vi "process data.vi"(0 "waveform array":waveform(dbl)[](array[waveform]), 11 "error in":errorcluster) -> (4 "device 1":cluster{"V":dbl, "dV":dbl, "Q":dbl, "dQ":dbl}, 6 "device 2":cluster{"V":dbl, "dV":dbl, "Q":dbl, "dQ":dbl}, 15 "error out":errorcluster)   [LabVIEW 2026]
uses:
  <vilib>/Utility/error.llb/Error Cluster From Error Code.vi
  <vilib>/ErrorRing/Error Ring.xnode
  <vilib>/Analysis/NI_AALBase.lvlib
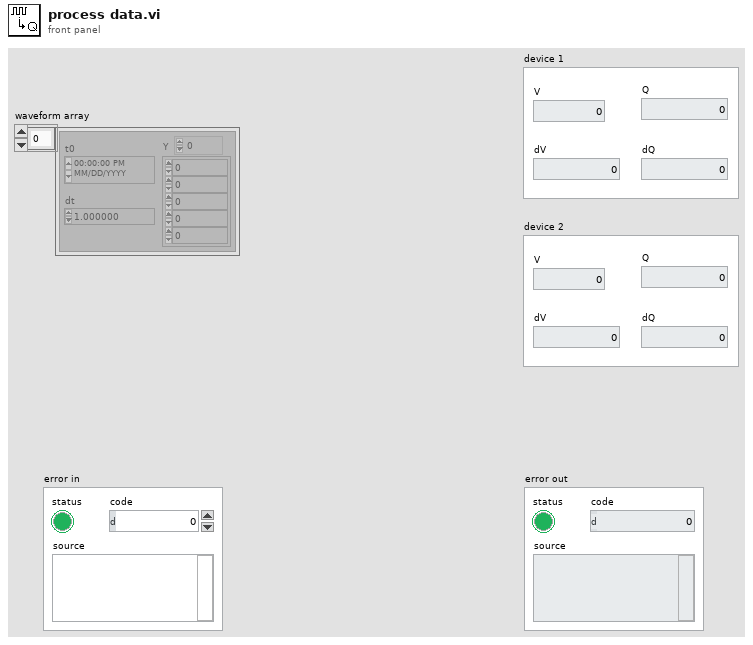
[diagram p1: front panel]
types:
  T1 = cluster{"waveform array[0]":waveform(dbl), "waveform array[1]":waveform(dbl), "waveform array[2]":waveform(dbl), "waveform array[3]":waveform(dbl), "waveform array[4]":waveform(dbl), "waveform array[5]":waveform(dbl), "waveform array[6]":waveform(dbl), "waveform array[7]":waveform(dbl), "waveform array[8]":waveform(dbl)}
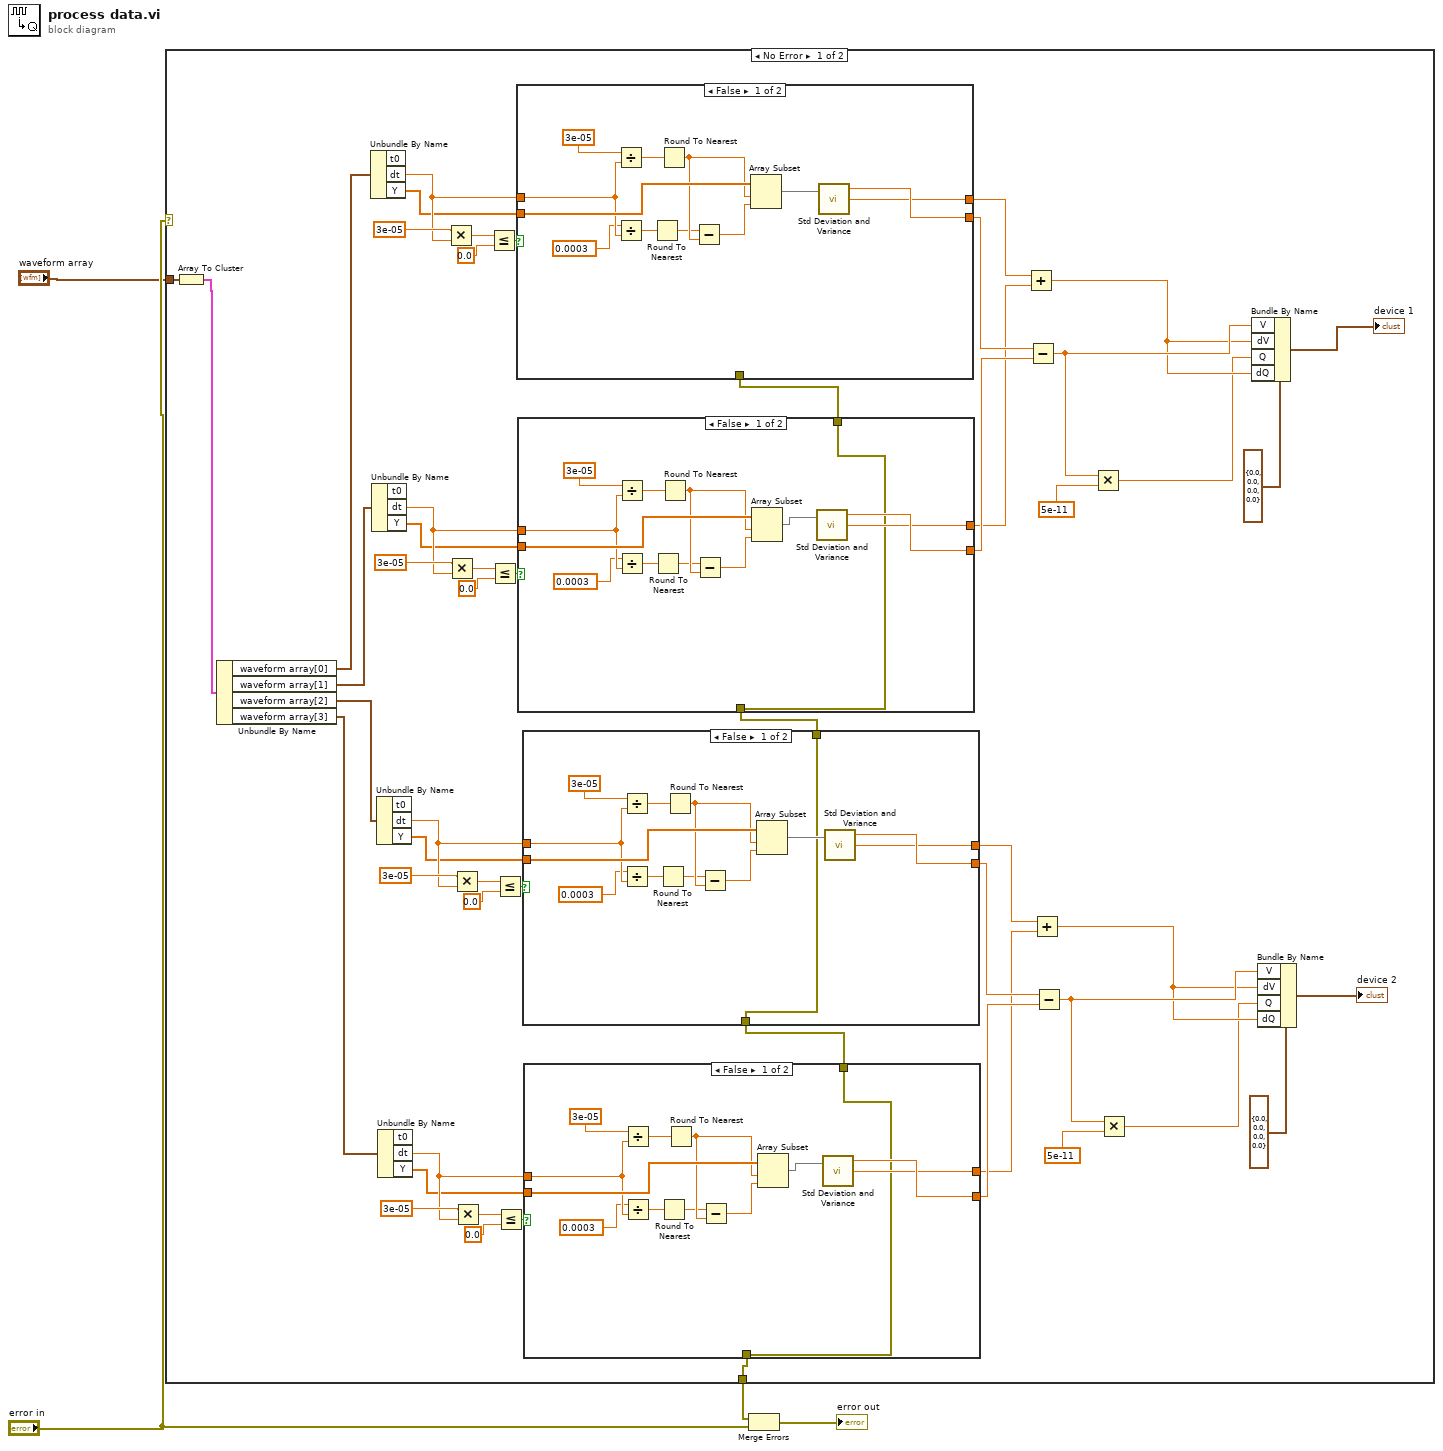
[diagram p0: block diagram]
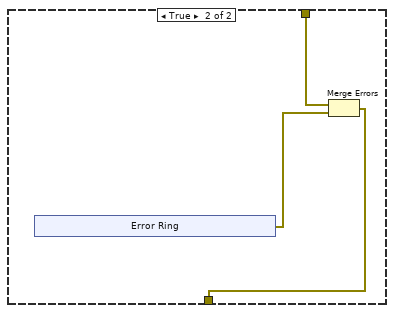
[diagram p2: hidden frame]
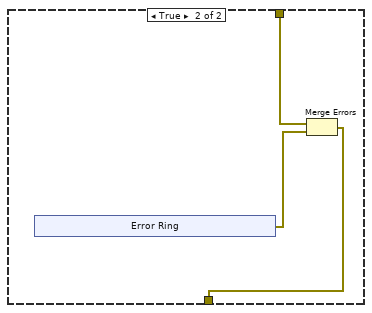
[diagram p3: hidden frame]
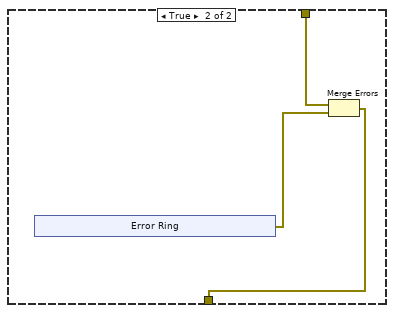
[diagram p4: hidden frame]
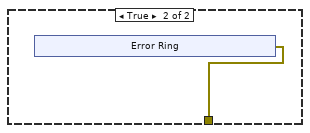
[diagram p5: hidden frame]
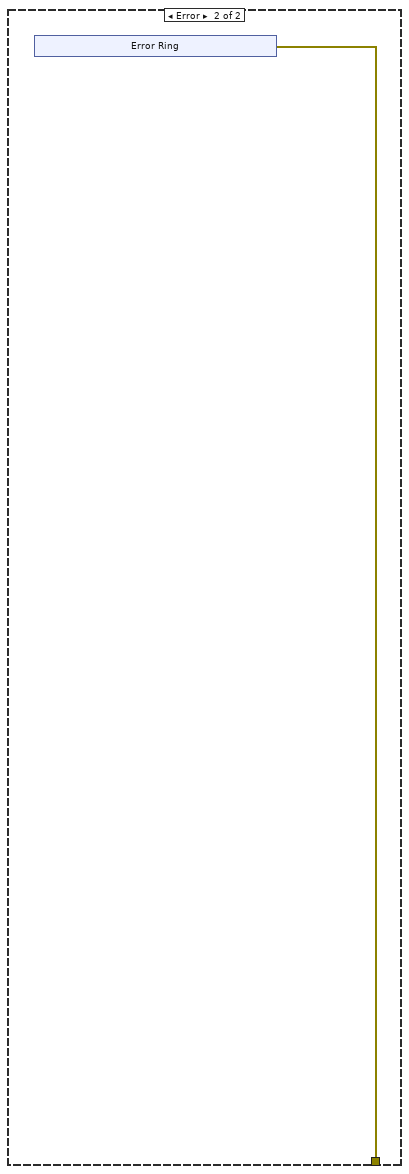
[diagram p6: hidden frame]
diagram:
  n1 = case shown="No Error" "error in" {
    tunnel: "waveform array" -> [w52 _]
    tunnel: [w5 w140] -> w3
    frame No Error {
      n2 = Array To Cluster(array=w52) -> (cluster=w51:T1)
      n3 = Unbundle By Name(w51) -> ("waveform array[0]"=w50:waveform(dbl), "waveform array[1]"=w43:waveform(dbl), "waveform array[2]"=w9:waveform(dbl), "waveform array[3]"=w8:waveform(dbl))
      n4 = Unbundle By Name(w50) -> ("dt"=w54:dbl, "Y"=w53:dbl[])  [unwired: 1 out]
      n5 = Unbundle By Name(w43) -> ("dt"=w45:dbl, "Y"=w44:dbl[])  [unwired: 1 out]
      n6 = Unbundle By Name(w9) -> ("dt"=w27:dbl, "Y"=w26:dbl[])  [unwired: 1 out]
      n7 = Unbundle By Name(w8) -> ("dt"=w21:dbl, "Y"=w20:dbl[])  [unwired: 1 out]
      n8 = Multiply(x=3e-05, y=w54) -> (x*y=w57:dbl)
      n9 = Multiply(x=3e-05, y=w45) -> (x*y=w48:dbl)
      n10 = Multiply(x=3e-05, y=w27) -> (x*y=w30:dbl)
      n11 = Multiply(x=3e-05, y=w21) -> (x*y=w24:dbl)
      n12 = Less Or Equal?(x=w57, y=0.0) -> (x <= y?=w55:bool)
      n13 = Less Or Equal?(x=w48, y=0.0) -> (x <= y?=w46:bool)
      n14 = Less Or Equal?(x=w30, y=0.0) -> (x <= y?=w28:bool)
      n15 = Less Or Equal?(x=w24, y=0.0) -> (x <= y?=w22:bool)
      n16 = case shown="False" w55 {
        tunnel: [_ w134] -> w37
        tunnel: w54 -> [w126 _]
        tunnel: w53 -> [w131 _]
        tunnel: [w123 _] -> w41
        tunnel: [w122 _] -> w39
        frame False {
          n17 = Divide(x=3e-05, y=w126) -> (x/y=w132:dbl)
          n18 = Divide(x=0.0003 ("y"), y=w126) -> (x/y=w128:dbl)
          n19 = Round To Nearest(number=w128) -> (nearest integer value=w127:dbl)
          n20 = Round To Nearest(number=w132) -> (nearest integer value=w129:dbl)
          n21 = Subtract(x=w127, y=w129) -> (x-y=w130:dbl)
          n22 = Array Subset(array=w131, index=w129, length=w130) -> (w124:dbl[])
          n23 = call <vilib>:"Std Deviation and Variance.vi"("X"=w124) -> ("mean"=w123:dbl, "standard deviation"=w122:dbl)  [unwired: 1 in, 1 out]
        }
        frame True {
          n24 = xnode "Error Ring"() -> ("error out"=w134:errorcluster)
        }
      }
      n25 = case shown="False" w46 {
        tunnel: [w101 w114] -> w6
        tunnel: w45 -> [w106 _]
        tunnel: w44 -> [w111 _]
        tunnel: [w103 _] -> w40
        tunnel: [w102 _] -> w38
        tunnel: w37 -> [w101 w116]
        frame False {
          n26 = Divide(x=3e-05, y=w106) -> (x/y=w112:dbl)
          n27 = Divide(x=0.0003 ("y"), y=w106) -> (x/y=w108:dbl)
          n28 = Round To Nearest(number=w108) -> (nearest integer value=w107:dbl)
          n29 = Round To Nearest(number=w112) -> (nearest integer value=w109:dbl)
          n30 = Subtract(x=w107, y=w109) -> (x-y=w110:dbl)
          n31 = Array Subset(array=w111, index=w109, length=w110) -> (w104:dbl[])
          n32 = call <vilib>:"Std Deviation and Variance.vi"("X"=w104) -> ("mean"=w103:dbl, "standard deviation"=w102:dbl)  [unwired: 1 in, 1 out]
        }
        frame True {
          n33 = xnode "Error Ring"() -> ("error out"=w115:errorcluster)
          n34 = Merge Errors(w116, w115) -> (w114:errorcluster)
        }
      }
      n35 = case shown="False" w28 {
        tunnel: [w80 w93] -> w14
        tunnel: w27 -> [w85 _]
        tunnel: w26 -> [w90 _]
        tunnel: [w82 _] -> w18
        tunnel: [w81 _] -> w16
        tunnel: w6 -> [w80 w95]
        frame False {
          n36 = Divide(x=3e-05, y=w85) -> (x/y=w91:dbl)
          n37 = Divide(x=0.0003 ("y"), y=w85) -> (x/y=w87:dbl)
          n38 = Round To Nearest(number=w87) -> (nearest integer value=w86:dbl)
          n39 = Round To Nearest(number=w91) -> (nearest integer value=w88:dbl)
          n40 = Subtract(x=w86, y=w88) -> (x-y=w89:dbl)
          n41 = Array Subset(array=w90, index=w88, length=w89) -> (w83:dbl[])
          n42 = call <vilib>:"Std Deviation and Variance.vi"("X"=w83) -> ("mean"=w82:dbl, "standard deviation"=w81:dbl)  [unwired: 1 in, 1 out]
        }
        frame True {
          n43 = xnode "Error Ring"() -> ("error out"=w94:errorcluster)
          n44 = Merge Errors(w95, w94) -> (w93:errorcluster)
        }
      }
      n45 = case shown="False" w22 {
        tunnel: [w59 w72] -> w5
        tunnel: w21 -> [w64 _]
        tunnel: w20 -> [w69 _]
        tunnel: [w61 _] -> w17
        tunnel: [w60 _] -> w15
        tunnel: w14 -> [w59 w74]
        frame False {
          n46 = Divide(x=3e-05, y=w64) -> (x/y=w70:dbl)
          n47 = Divide(x=0.0003 ("y"), y=w64) -> (x/y=w66:dbl)
          n48 = Round To Nearest(number=w66) -> (nearest integer value=w65:dbl)
          n49 = Round To Nearest(number=w70) -> (nearest integer value=w67:dbl)
          n50 = Subtract(x=w65, y=w67) -> (x-y=w68:dbl)
          n51 = Array Subset(array=w69, index=w67, length=w68) -> (w62:dbl[])
          n52 = call <vilib>:"Std Deviation and Variance.vi"("X"=w62) -> ("mean"=w61:dbl, "standard deviation"=w60:dbl)  [unwired: 1 in, 1 out]
        }
        frame True {
          n53 = xnode "Error Ring"() -> ("error out"=w73:errorcluster)
          n54 = Merge Errors(w74, w73) -> (w72:errorcluster)
        }
      }
      n55 = Add(x=w39, y=w38) -> (x+y=w34:dbl)
      n56 = Subtract(x=w41, y=w40) -> (x-y=w35:dbl)
      n57 = Add(x=w16, y=w15) -> (x+y=w11:dbl)
      n58 = Subtract(x=w18, y=w17) -> (x-y=w12:dbl)
      n59 = Multiply(x=w35, y=5e-11) -> (x*y=w33:dbl)
      n60 = Multiply(x=w12, y=5e-11) -> (x*y=w10:dbl)
      n61 = Bundle By Name(cluster=cluster{"V":dbl, "dV":dbl, "Q":dbl, "dQ":dbl} {"V"=0.0, "dV"=0.0, "Q"=0.0, "dQ"=0.0} ("device 1"), "V"=w35, "dV"=w34, "Q"=w33, "dQ"=w34) -> (→"device 1":cluster{"V":dbl, "dV":dbl, "Q":dbl, "dQ":dbl})
      n62 = Bundle By Name(cluster=cluster{"V":dbl, "dV":dbl, "Q":dbl, "dQ":dbl} {"V"=0.0, "dV"=0.0, "Q"=0.0, "dQ"=0.0} ("device 1"), "V"=w12, "dV"=w11, "Q"=w10, "dQ"=w11) -> (→"device 2":cluster{"V":dbl, "dV":dbl, "Q":dbl, "dQ":dbl})
    }
    frame Error {
      n63 = xnode "Error Ring"() -> ("error out"=w140:errorcluster)
    }
  }
  n64 = Merge Errors(w3, "error in") -> (→"error out":errorcluster)
